vi "Get Default Save Folder Path.vi"() -> (3 "Path":path)   [LabVIEW 2020, in "Process Generation.lvlib" / "New Class Dialog.lvclass"]
uses:
  New Class Dialog.lvclass
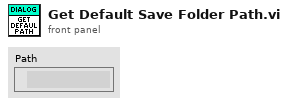
[diagram p1: front panel]
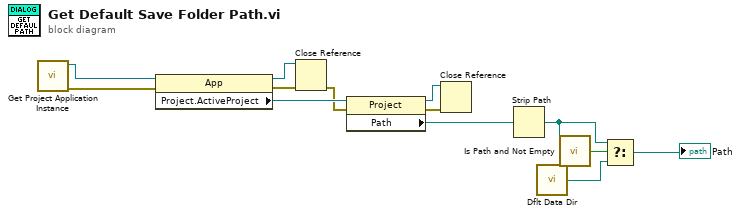
[diagram p0: block diagram]
diagram:
  n1 = call "Get Project Application Instance.vi"() -> ("error out"=w12:errorcluster, "Application out"=w13:refnum<vi>)  [unwired: 10 in]
  n2 = property class="App"(reference=w13, error in=w12) -> (reference out=w10:refnum<vi>, error out=w11:errorcluster, "Project.ActiveProject"=w9:refnum<vi>)
  n3 = Close Reference(reference=w10, error in (no error)=w11) -> (error out=w8:errorcluster)
  n4 = property class="Project"(reference=w9, error in=w8) -> (reference out=w6:refnum<vi>, error out=w7:errorcluster, "Path"=w5:path)
  n5 = Close Reference(reference=w6, error in (no error)=w7) -> ()  [unwired: 1 out]
  n6 = Strip Path(path=w5) -> (stripped path=w3:path)  [unwired: 1 out]
  n7 = call <vilib>:"Dflt Data Dir.vi"() -> ("App:Default Data Directory"=w1:path)
  n8 = call <vilib>:"Is Path and Not Empty.vi"("path"=w3) -> ("Is Path and Not Empty?"=w4:bool)  [unwired: 4 in]
  n9 = Select(t=w3, s=w4, f=w1) -> (s? t:f=→"Path":path)
